vi "Get XY Coordinates.vi"() -> (0 "Y":dbl, 1 "X":dbl)   [LabVIEW 2018]
uses:
  Robot Global Data.vi
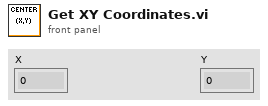
[diagram p1: front panel]
types:
  T1 = cluster{"Distance (ft)":dbl, "Score":dbl, "Normalized":cluster{"Center":cluster{dbl, dbl}, "Rectangle":cluster{"Numeric":dbl, "Numeric 2":dbl, "Numeric 3":dbl, "Numeric 5":dbl}}, "Pixels":cluster{"Center":cluster{dbl, dbl}, "Rectangle":cluster{"Numeric":dbl, "Numeric 2":dbl, "Numeric 3":dbl, "Numeric 5":dbl}}}
  T2 = cluster{"Center":cluster{dbl, dbl}, "Rectangle":cluster{"Numeric":dbl, "Numeric 2":dbl, "Numeric 3":dbl, "Numeric 5":dbl}}
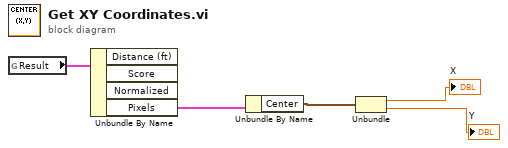
[diagram p0: block diagram]
diagram:
  n1 = global read "Robot Global Data.vi" "Result"() -> (w5:T1)
  n2 = Unbundle By Name(w5) -> ("Pixels"=w4:T2)  [unwired: 3 out]
  n3 = Unbundle By Name(w4) -> ("Center"=w3:cluster{dbl, dbl})
  n4 = Unbundle(w3) -> (→"X":dbl, →"Y":dbl)
